vi "NewPath.xio.vi"(8 "Append path":string, 9 "Basic path":path) -> (3 "New path":path)   [LabVIEW 2018]
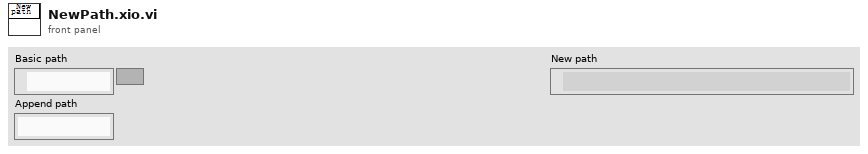
[diagram p1: front panel]
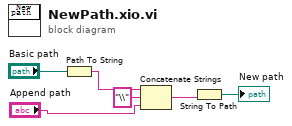
[diagram p0: block diagram]
diagram:
  n1 = Path To String(path="Basic path") -> (string=w5:string)
  n2 = Concatenate Strings(w5, "\\" ("字符串"), "Append path") -> (w4:string)
  n3 = String To Path(string=w4) -> (path=→"New path":path)
